vi "util.numToRoundString.vi"(10 "precision(1)":i16=1, 11 "reg in":dbl) -> (3 "String":string)   [LabVIEW 2024]
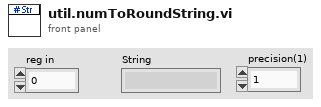
[diagram p1: front panel]
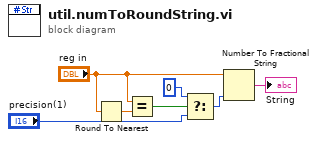
[diagram p0: block diagram]
diagram:
  n1 = Round To Nearest(number="reg in") -> (nearest integer value=w2:dbl)
  n2 = Equal?(x="reg in", y=w2) -> (x = y?=w3:bool)
  n3 = Select(t=i16 0 ("width (-)"), s=w3, f="precision(1)") -> (s? t:f=w6:i16)
  n4 = Number To Fractional String(number="reg in", precision (6)=w6) -> (F-format string=→"String":string)  [unwired: 2 in]
